vi "OAT Polar angle labels.vi"(5 "[user-specified font]":T3, 7 "desired font(Application)":T2(ring)=enum."Application Font", 8 "shaft rotating direction":u16(ring) items=["CCW", "CW"], 9 "grid measurements":T1={"pixel center"={"x"=175, "y"=175}, "scale factors"={"a"=7195.980240002514, "b"=0.0, "log?"=FALSE}, "grid color"=3381657, "start angle"=0.0, "end angle"=360.0, "tick length"=159, "pixel radius"=157} {"end angle" format="%.2f"; "start angle" format="%.2f"; "scale factors"."b" format="%.2f"; "scale factors"."a" format="%.2f"}, 10 "probe position":u16, 11 "picture":picture) -> (3 "new picture":picture)   [LabVIEW 2017]
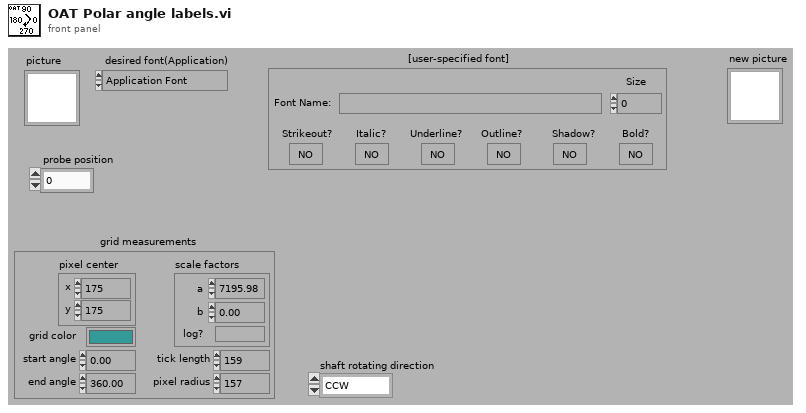
[diagram p1: front panel]
types:
  T1 = cluster{"pixel center":cluster{"x":i16, "y":i16}, "scale factors":cluster{"a":dbl, "b":dbl, "log?":bool}, "grid color":u32, "start angle":dbl, "end angle":dbl, "tick length":i16, "pixel radius":i32}
  T2 = enum16{"User-specified Font", "Application Font", "System Font", "Dialog Font"}
  T3 = cluster{"Font Name:":string, "Size":i16, "Strikeout?":bool, "Italic?":bool, "Underline?":bool, "Outline?":bool, "Shadow?":bool, "Bold?":bool}
  T4 = cluster{"horizontal":enum16{"left", "center", "right"}, "vertical":enum16{"top", "center", "bottom"}}[]
  T5 = cluster{"horizontal":enum16{"left", "center", "right"}, "vertical":enum16{"top", "center", "bottom"}}
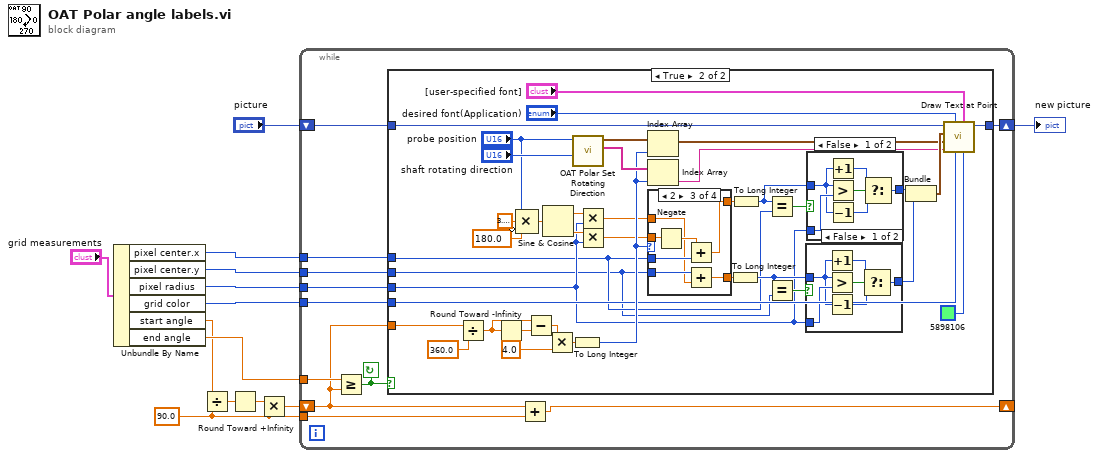
[diagram p0: block diagram]
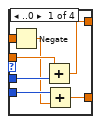
[diagram p5: hidden frame]
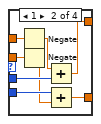
[diagram p6: hidden frame]
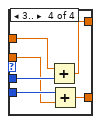
[diagram p7: hidden frame]
diagram:
  w6 = 90.0
  n1 = Unbundle By Name("grid measurements") -> ("pixel center.x"=w1:i16, "pixel center.y"=w2:i16, "pixel radius"=w3:i32, "grid color"=w10:u32, "start angle"=w4:dbl, "end angle"=w5:dbl)
  n2 = Divide(x=w4, y=w6) -> (x/y=w9:dbl)
  n3 = Round Toward +Infinity(x=w9) -> (ceil(x): smallest int >= x=w8:dbl)
  n4 = Multiply(x=w8, y=w6) -> (x*y=w7:dbl)
  n5 = while {
    tunnel: w10 -> [w14]
    tunnel: w1 -> [w15]
    tunnel: w2 -> [w16]
    tunnel: w3 -> [w17]
    shift-left: "picture" -> [w18]
    shift-right: [w19] -> w12
    tunnel: w5 -> [w23]
    tunnel: w6 -> [w24]
    shift-left: w7 -> [w20]
    shift-right: [w22] -> _
    stop <- w21 continue-if-true
    n6 = Greater Or Equal?(x=w23, y=w20) -> (x >= y?=w21:bool)
    n7 = case shown="True" w21 {
      tunnel: w20 -> [_ w59]
      tunnel: [w25 w57] -> w19
      tunnel: w18 -> [w25 w56]
      tunnel: w17 -> [_ w29]
      tunnel: w16 -> [_ w27]
      tunnel: w15 -> [_ w28]
      tunnel: w14 -> [_ w30]
      frame False {
      }
      frame True {
        n8 = Divide(x=w59, y=360.0) -> (x/y=w62:dbl)
        n9 = Round Toward -Infinity(1:w62) -> (0:w61:dbl)
        n10 = Compound Arithmetic op=MULTIPLY("probe position", 3.141592653589793, invert 180.0 ("value")) -> (w42:dbl)
        n11 = Subtract(x=w62, y=w61) -> (x-y=w63:dbl)
        n12 = Sine & Cosine(0:w42) -> (1:w41:dbl, 2:w40:dbl)
        n13 = Multiply(x=w63, y=4.0) -> (x*y=w52:dbl)
        n14 = To Long Integer(number=w52) -> (32bit integer=w46:i32)
        n15 = call <vilib>:"OAT Polar Set Rotating Direction.vi"("shaft rotating direction"="shaft rotating direction", "probe position"="probe position") -> ("label out"=w50:string[], "label justification"=w47:T4)  [unwired: 7 in, 1 out]
        n16 = Multiply(x=w41, y=w29) -> (x*y=w26:dbl)
        n17 = Multiply(x=w40, y=w29) -> (x*y=w39:dbl)
        n18 = Index Array(array=w47, index=w46) -> (element=w51:T5)
        n19 = Index Array(array=w50, index=w46) -> (element=w53:string)
        n20 = case shown="2" w46 {
          tunnel: [w81 w88 w98 w103] -> w38
          tunnel: [w80 w87 w97 w102] -> w37
          tunnel: w28 -> [w85 w93 w100 w106]
          tunnel: w27 -> [w84 w91 w99 w104]
          tunnel: w26 -> [w82 w92 w94 w105]
          tunnel: w39 -> [w83 w90 w96 w101]
          frame ..0 {
            n21 = Negate(x=w82) -> (-x=w79:dbl)
            n22 = Add(x=w83, y=w85) -> (x+y=w81:dbl)
            n23 = Add(x=w84, y=w79) -> (x+y=w80:dbl)
          }
          frame 1 {
            n24 = Negate(x=w92) -> (-x=w89:dbl)
            n25 = Negate(x=w90) -> (-x=w86:dbl)
            n26 = Add(x=w89, y=w93) -> (x+y=w88:dbl)
            n27 = Add(x=w91, y=w86) -> (x+y=w87:dbl)
          }
          frame 2 {
            n28 = Negate(x=w96) -> (-x=w95:dbl)
            n29 = Add(x=w95, y=w100) -> (x+y=w98:dbl)
            n30 = Add(x=w99, y=w94) -> (x+y=w97:dbl)
          }
          frame 3.. {
            n31 = Add(x=w105, y=w106) -> (x+y=w103:dbl)
            n32 = Add(x=w104, y=w101) -> (x+y=w102:dbl)
          }
        }
        n33 = To Long Integer(number=w37) -> (32bit integer=w31:i32)
        n34 = To Long Integer(number=w38) -> (32bit integer=w35:i32)
        n35 = Equal?(x=w35, y=w28) -> (x = y?=w36:bool)
        n36 = Equal?(x=w31, y=w27) -> (x = y?=w33:bool)
        n37 = case shown="False" w33 {
          tunnel: w31 -> [w66 w71]
          tunnel: [w65 w71] -> w32
          tunnel: w29 -> [w68 _]
          frame False {
            n38 = Increment(x=w66) -> (x+1=w70:i32)
            n39 = Greater?(x=w66, y=w68) -> (0:w67:bool)
            n40 = Decrement(x=w66) -> (x-1=w69:i32)
            n41 = Select(t=w70, s=w67, f=w69) -> (s? t:f=w65:i32)
          }
          frame True {
          }
        }
        n42 = case shown="False" w36 {
          tunnel: w35 -> [w73 w78]
          tunnel: [w72 w78] -> w34
          tunnel: w29 -> [w75 _]
          frame False {
            n43 = Increment(x=w73) -> (x+1=w77:i32)
            n44 = Greater?(x=w73, y=w75) -> (0:w74:bool)
            n45 = Decrement(x=w73) -> (x-1=w76:i32)
            n46 = Select(t=w77, s=w74, f=w76) -> (s? t:f=w72:i32)
          }
          frame True {
          }
        }
        n47 = Bundle(w34, w32) -> (w58:cluster{i32, i32})  [unwired: 1 in]
        n48 = call <vilib>:"Draw Text at Point.vi"("BG color(transparent)"=u32 5898106, "[user-specified font]"="[user-specified font]", "text color(black)"=w30, "desired font(Application)"="desired font(Application)", "text"=w53, "alignment(left, top)"=w51, "origin"=w58, "picture"=w56) -> ("new picture"=w57:picture)  [unwired: 2 in, 1 out]
      }
    }
    n49 = Add(x=w20, y=w24) -> (x+y=w22:dbl)
  }
  "new picture" <- w12
